vi "Matrix RGB.vi"() -> ()   [LabVIEW 2019]
uses:
  LED Matrix Host/Public/Controls/Animation.ctl
  <vilib>/FPGAPlugInAG/myRIO-1900/niLvFpga_Open_myRIO-1900.vi
  <vilib>/rvi/interface/common/dynamic/niFpgaDynamicAddResources.vi
  <vilib>/Utility/error.llb/Error Cluster From Error Code.vi
  <vilib>/rvi/errors/niLvFpgaAdjustHostInterfaceError.vi
  <vilib>/FPGAPlugInAG/Dynamic/niLvFpga_Close_Dynamic.vi
  <vilib>/rvi/interface/nirviOpenFPGA/nirviOpenFPGA.xnode
  FPGA Bitfiles/ledmatrix_FPGATarget_MainFPGA_p8SXomXGKcI.lvbitx
  <vilib>/rvi/interface/nirviReadWriteControl/nirviReadWriteControl.xnode
  <vilib>/rvi/interface/nirviCloseFPGA/nirviCloseFPGA.xnode
  NiFpgaLv.dll
  <vilib>/rvi/interface/Simulation/niFpgaSimulationCallBeginRW.vi
  LED Matrix Host/LED Matrix Host.lvlib
panel:
  in  "Color Box":u32(colorbox)=6618880
  in  "Tab Control":enum32{"Matrix Manual", "Animation", "Control"}(tab)
  in  "Matrix":u32[][](array[colorbox])
  in  "Animation":T1
  in  "Tank":u8(slide) max=8 scale=0.0..8.0
  in  "FPS":u32(slide) scale=0.0..100.0
  in  "Update":bool
  in  "stop":bool
  in  "Intensity":sgl(slide) scale=0.0..1.0
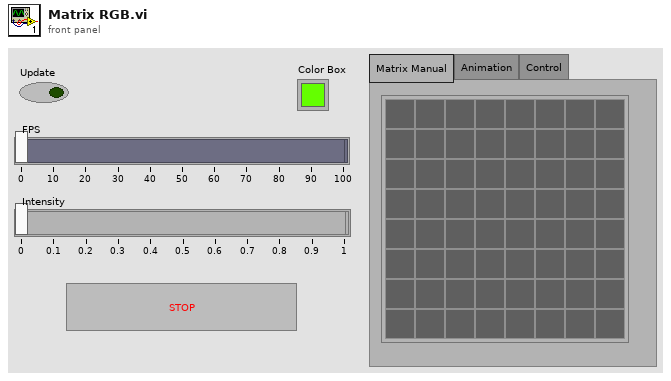
[diagram p1: front panel]
types:
  T1 = typedef "LED Matrix Host.lvlib/Animation.ctl" = enum16{"Pixel Pass", "Columns Pass", "Rows Pass", "Frame Pass"}
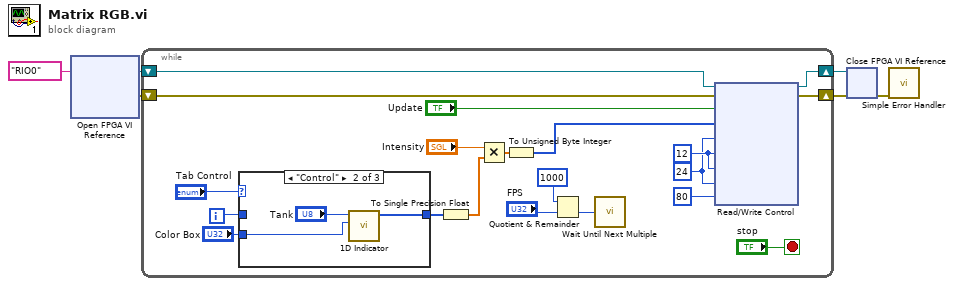
[diagram p0: block diagram]
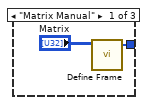
[diagram p2: hidden frame]
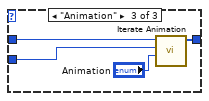
[diagram p3: hidden frame]
diagram:
  n1 = xnode "Open FPGA VI Reference"("resource name"=tag "RIO0") -> ("FPGA VI Reference Out"=w5:refnum<k20>, "error out"=w4:errorcluster)  [unwired: 1 in]
  n2 = while {
    shift-right: [w23] -> w3
    shift-left: w5 -> [w26]
    shift-right: [w22] -> w2
    shift-left: w4 -> [w25]
    i -> [w11]
    stop <- "stop" stop-if-true
    w18 = u8 12 ("High False")
    w17 = u8 24 ("High True")
    n3 = case shown="\"Control\"" "Tab Control" {
      tunnel: [w28 w29 w35] -> w10
      tunnel: w11 -> [_ _ w34]
      tunnel: "Color Box" -> [_ w30 w32]
      frame "Matrix Manual" {
        n4 = call "Define Frame.vi"("Matrix"="Matrix") -> ("Array"=w28:u8[])  [unwired: 10 in]
      }
      frame "Control" {
        n5 = call "1D Indicator.vi"("Color"=w30, "Numeric Value"="Tank") -> ("Raw Data"=w29:u8[])  [unwired: 9 in]
      }
      frame "Animation" {
        n6 = call "Iterate Animation.vi"("Animation"="Animation", "Color"=w32, "Index"=w34) -> ("Raw Data"=w35:u8[])  [unwired: 8 in]
      }
    }
    n7 = To Single Precision Float(number=w10) -> (single precision float=w15:sgl[])
    n8 = Multiply(x="Intensity", y=w15) -> (x*y=w16:sgl[])
    n9 = To Unsigned Byte Integer(number=w16) -> (unsigned 8bit integer=w9:u8[])
    n10 = Quotient & Remainder(x=u32 1000 ("y"), y="FPS") -> (floor(x/y)=w12:u32)  [unwired: 1 out]
    n11 = call "Wait Until Next Multiple"("Count(mSec)"=w12) -> ()  [unwired: 1 out]
    n12 = xnode "Read/Write Control"("FPGA VI Reference In"=w26, "error in"=w25, "Update"="Update", "Matrix Array"=w9, "High True"=w17, "High False"=w18, "Low True"=w18, "Low False"=w17, "Reset (us)"=u16 80 ("Reset")) -> ("FPGA VI Reference Out"=w23:refnum<k20>, "error out"=w22:errorcluster)
  }
  n13 = xnode "Close FPGA VI Reference"("FPGA VI Reference In"=w3, "error in"=w2) -> ("error out"=w1:errorcluster)
  n14 = call <vilib>:"Simple Error Handler.vi"("error in (no error)"=w1) -> ()  [unwired: 4 in, 5 out]
